vi "Write On.vi"(8 "error in (no error)":errorcluster, 10 "On":bool, 11 "PSU in":refnum<class "PSU.lvclass">) -> (0 "error out":errorcluster, 3 "PSU out":refnum<class "PSU.lvclass">)   [LabVIEW 2014, in "PSU.lvclass"]
uses:
  PSU.lvclass
  PSU.lvclass/PSU.ctl
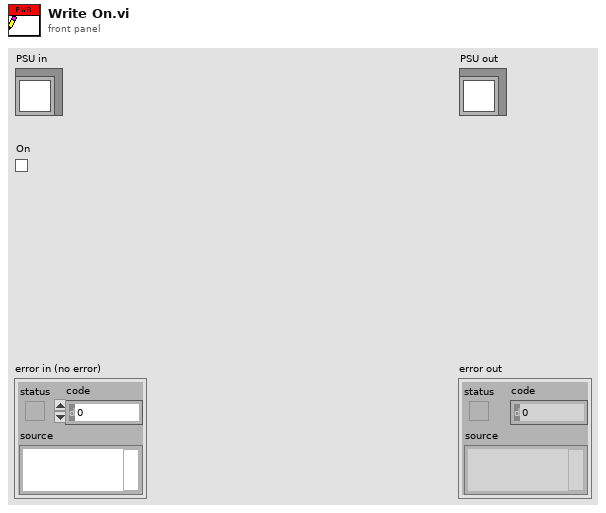
[diagram p1: front panel]
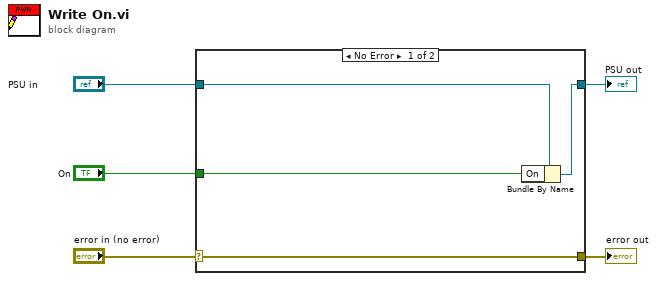
[diagram p0: block diagram]
diagram:
  n1 = case shown="No Error" "error in (no error)" {
    selector: "error in (no error)" -> [w9 w10]
    tunnel: [w9 w10] -> w4
    tunnel: [w7 w11] -> w2
    tunnel: "PSU in" -> [w8 w11]
    tunnel: "On" -> [w6 _]
    frame No Error {
      n2 = Bundle By Name(cluster=w8, "On"=w6) -> (w7:refnum<class "PSU.lvclass">)
    }
    frame Error {
    }
  }
  "error out" <- w4
  "PSU out" <- w2
